vi "Translator AD9850.vi"() -> ()   [LabVIEW 2014, in "LabVIEW Universal Transcriptor AD9850.lvlib" / "AD9850.lvclass"]
uses:
  AD9850.lvclass
panel:
  out "Outputs":string[](array[string])
  out "Inputs":string[](array[string])
  out "Output Datatypes":string[](array[string])
  out "Input Datatypes":string[](array[string])
  out "Output":variant=variant("Defines"=variant(string[] []), "Includes"=variant(string[] []), "Replaced Code"=variant(string "/* LabVIEW system function 'Strip Path' not found. */"))
  in  "Input":variant=variant("Function Name"=variant(string "Strip Path"), "Input Datatypes"=variant(string[] ["error", "int"]), "Inputs"=variant(string[] ["error in", "x"]), "Node refnum"=variant(refnum<vi> refnum), "Output Datatypes"=variant(string[] ["int"]), "Outputs"=variant(string[] ["a"]))
  out "error out":errorcluster
  in  "error in (no error)":errorcluster
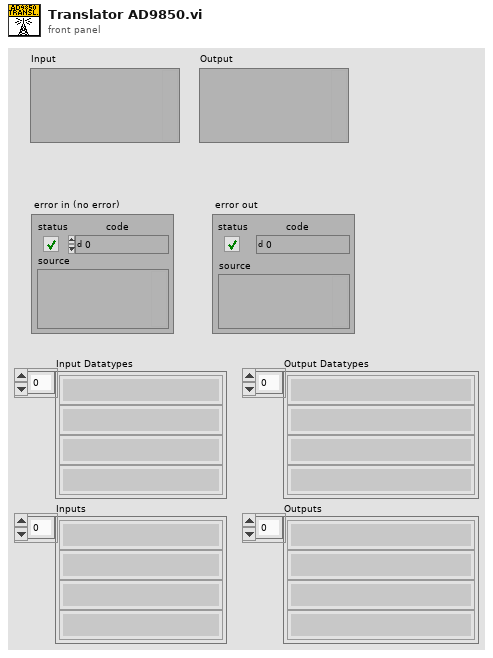
[diagram p1: front panel]
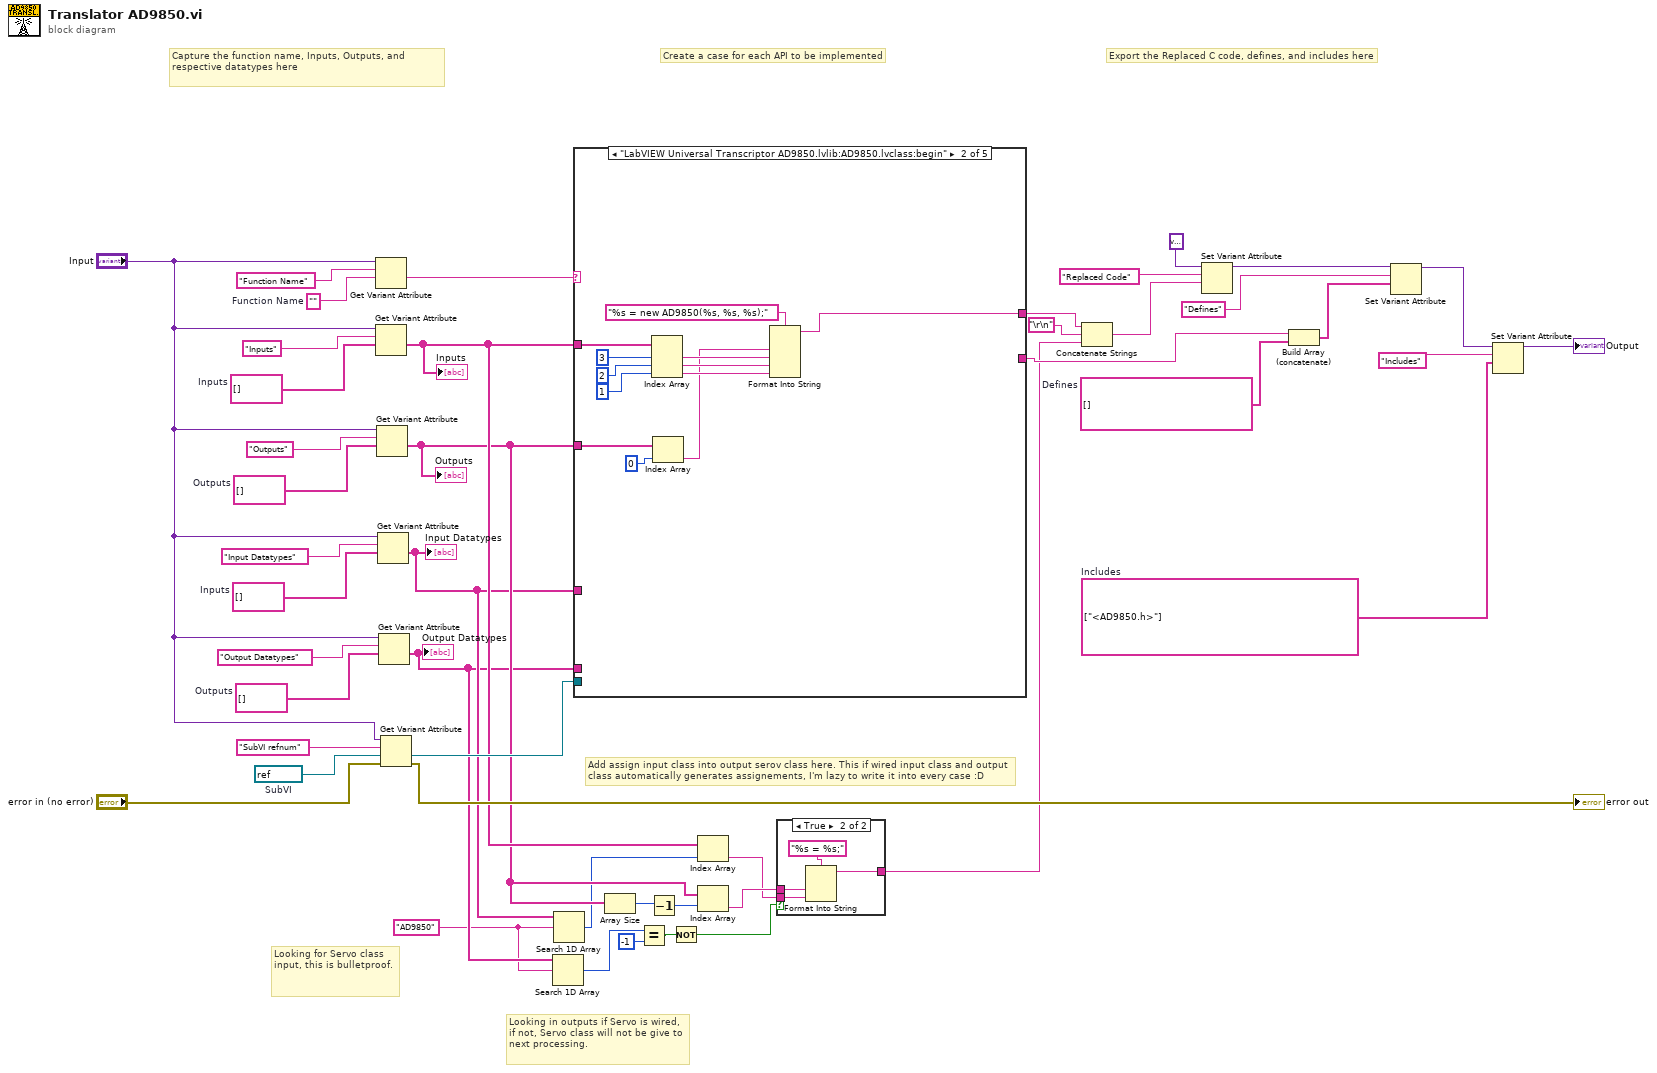
[diagram p0: block diagram]
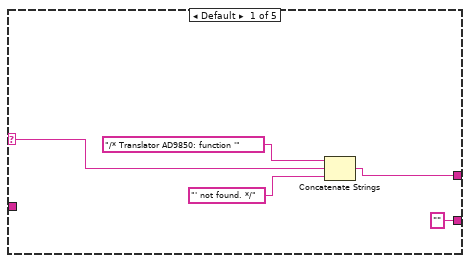
[diagram p3: hidden frame]
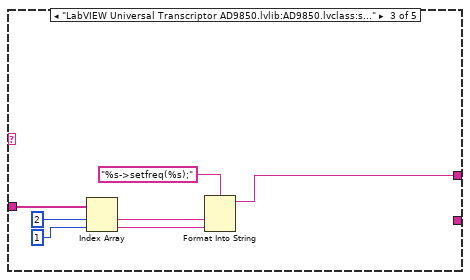
[diagram p4: hidden frame]
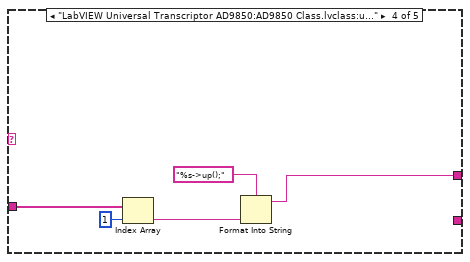
[diagram p5: hidden frame]
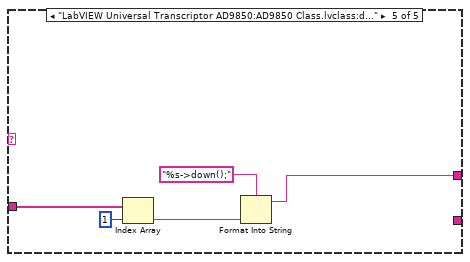
[diagram p6: hidden frame]
diagram:
  w2 = "AD9850" ("format string")
  w26 = refnum<vi> refnum  # SubVI
  w21 = string[] []  # Defines
  w33 = string[] []  # Outputs
  w34 = string[] []  # Inputs
  w24 = string[] ["<AD9850.h>"]  # Includes
  w42 = string[] []  # Outputs
  w43 = string[] []  # Inputs
  w44 = ""  # Function Name
  # "Looking for Servo class input, this is bulletproof."
  # "Looking in outputs if Servo is wired, if not, Servo class will not be give to next processing."
  # "Add assign input class into output serov class here. This if wired input class and output class automatically generates assignements, I'm lazy to write it into every case :D"
  # "Capture the function name, Inputs, Outputs, and respective datatypes here"
  # "Export the Replaced C code, defines, and includes here"
  # "Create a case for each API to be implemented"
  n1 = Get Variant Attribute(Variant="Input", name="Function Name", default value (empty Variant)=w44) -> (value=w39:string)  [unwired: 1 in, 3 out]
  n2 = Get Variant Attribute(Variant="Input", name="Inputs", default value (empty Variant)=w43) -> (value=w10:string[])  [unwired: 1 in, 3 out]
  "Inputs" <- w10
  n3 = Get Variant Attribute(Variant="Input", name="Outputs", default value (empty Variant)=w42) -> (value=w9:string[])  [unwired: 1 in, 3 out]
  "Outputs" <- w9
  n4 = Get Variant Attribute(Variant="Input", name="Input Datatypes", default value (empty Variant)=w34) -> (value=w8:string[])  [unwired: 1 in, 3 out]
  "Input Datatypes" <- w8
  n5 = Get Variant Attribute(Variant="Input", name="Output Datatypes", default value (empty Variant)=w33) -> (value=w3:string[])  [unwired: 1 in, 3 out]
  "Output Datatypes" <- w3
  n6 = Get Variant Attribute(Variant="Input", name="SubVI refnum", default value (empty Variant)=w26, error in="error in (no error)") -> (value=w25:refnum<vi>, error out=→"error out":errorcluster)  [unwired: 2 out]
  n7 = Search 1D Array(1D array=w3, element=w2) -> (index of element=w1:i32)  [unwired: 1 in]
  n8 = Search 1D Array(1D array=w8, element=w2) -> (index of element=w6:i32)  [unwired: 1 in]
  n9 = case shown="\"LabVIEW Universal Transcriptor AD9850.lvlib:AD9850.lvclass:begin\"" w39 {
    selector: w39 -> [w50 _ _ _ _]
    tunnel: [w48 w55 w64 w71 w76] -> w14
    tunnel: w10 -> [_ w62 w69 w72 w77]
    tunnel: w9 -> [_ w54 _ _ _]
    tunnel: w8 -> [_ _ _ _ _]
    tunnel: w25 -> [_ _ _ _ _]
    tunnel: w3 -> [_ _ _ _ _]
    tunnel: ["" _ _ _ _] -> w19
    frame Default {
      n10 = Concatenate Strings("/* Translator AD9850: function '", w50, "' not found. */") -> (w48:string)
    }
    frame "LabVIEW Universal Transcriptor AD9850.lvlib:AD9850.lvclass:begin" {
      n11 = Index Array(array=w62, index #1=3 ("index"), index #2=2 ("index"), index #3=1 ("index")) -> (element #1=w61:string, element #2=w57:string, element #3=w56:string)
      n12 = Index Array(array=w54, index=0) -> (element=w52:string)
      n13 = Format Into String(format string="%s = new AD9850(%s, %s, %s);", w52, w61, w57, w56) -> (resulting string=w55:string)  [unwired: 2 in, 1 out]
    }
    frame "LabVIEW Universal Transcriptor AD9850.lvlib:AD9850.lvclass:setfreq" {
      n14 = Index Array(array=w69, index #1=2 ("index"), index #2=1 ("index")) -> (element #1=w68:string, element #2=w65:string)
      n15 = Format Into String(format string="%s->setfreq(%s);", w68, w65) -> (resulting string=w64:string)  [unwired: 2 in, 1 out]
    }
    frame "LabVIEW Universal Transcriptor AD9850:AD9850 Class.lvclass:up" {
      n16 = Index Array(array=w72, index=1) -> (element=w74:string)
      n17 = Format Into String(format string="%s->up();", w74) -> (resulting string=w71:string)  [unwired: 2 in, 1 out]
    }
    frame "LabVIEW Universal Transcriptor AD9850:AD9850 Class.lvclass:down" {
      n18 = Index Array(array=w77, index=1) -> (element=w79:string)
      n19 = Format Into String(format string="%s->down();", w79) -> (resulting string=w76:string)  [unwired: 2 in, 1 out]
    }
  }
  n20 = Array Size(array=w9) -> (size(s)=w18:i32)
  n21 = Equal?(x=w1, y=-1 ("index of element")) -> (x = y?=w5:bool)
  n22 = Decrement(x=w18) -> (x-1=w17:i32)
  n23 = Not(x=w5) -> (.not. x?=w4:bool)
  n24 = Index Array(array=w10, index=w6) -> (element=w15:string)
  n25 = Index Array(array=w9, index=w17) -> (element=w16:string)
  n26 = case shown="True" w4 {
    tunnel: w16 -> [_ w83]
    tunnel: w15 -> [_ w82]
    tunnel: [_ w81] -> w11
    frame False {
    }
    frame True {
      n27 = Format Into String(format string="%s = %s;", w83, w82) -> (resulting string=w81:string)  [unwired: 2 in, 1 out]
    }
  }
  n28 = Concatenate Strings(w14, "\r\n", w11) -> (w13:string)
  n29 = Set Variant Attribute(Variant=variant ("variant"), name="Replaced Code", value=w13) -> (Variant out=w31:variant)  [unwired: 1 in, 2 out]
  n30 = Build Array (concatenate)(w19, w21) -> (w20:string[])
  n31 = Set Variant Attribute(Variant=w31, name="Defines", value=w20) -> (Variant out=w30:variant)  [unwired: 1 in, 2 out]
  n32 = Set Variant Attribute(Variant=w30, name="Includes", value=w24) -> (Variant out=→"Output":variant)  [unwired: 1 in, 2 out]
